vi "OCR_OCR.vi"(8 "Error":errorcluster, 11 "Image Data":T4) -> (0 "Error Out":errorcluster, 2 "Status Of Each Line Out":bool[](array[boolean]), 3 "Text Out":T6[](array[typedef]), 5 "Colors Out":T7, 7 "Icon Sizing Out":T1={"Rule"=enum."Static", "Header"=TRUE, "Rows"=5, "Width"=32, "Position"=enum."MID-CTR"} {"Rows" min=1 max=5 step=1; "Width" min=7 max=32 step=1})   [LabVIEW 2009]
doc: "Extract text data from image cluster"
uses:
  Controls/Cluster/Cluster_Icon Color Set.ctl
  Controls/Enum/ENUM_Frame Template Select.ctl
  Controls/String_Picture/STRING_Line Display.ctl
  Controls/Cluster/Cluster_Image Data.ctl
  Controls/Cluster/CLuster_Selectoin Box.ctl
  Controls/Cluster/Cluster_Sizing Data.ctl
  Controls/Enum/ENUM_Icon Sizing.ctl
  Controls/Enum/RBENUM_Icon Position.ctl
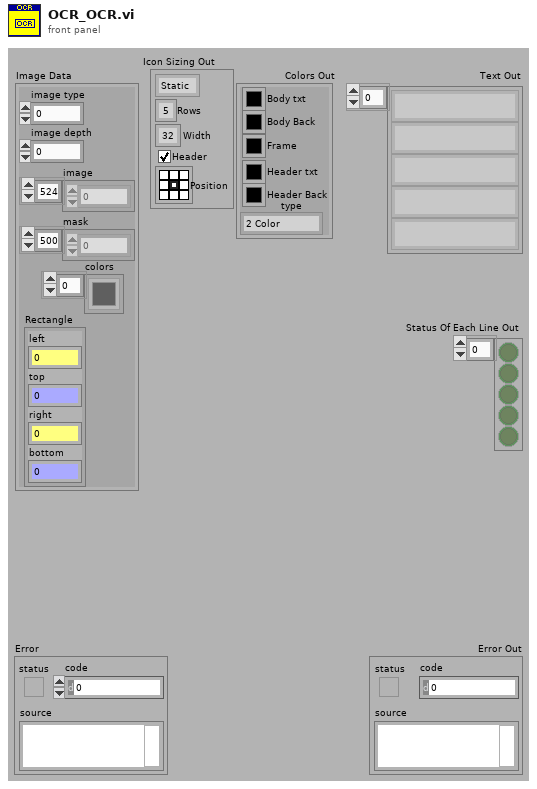
[diagram p1: front panel]
types:
  T1 = typedef "Cluster_Sizing Data.ctl" = cluster{"Rule":T2, "Header":bool, "Rows":u32, "Width":u32, "Position":T3}
  T2 = typedef "ENUM_Icon Sizing.ctl" = enum16{"Static", "Auto"}
  T3 = typedef "RBENUM_Icon Position.ctl" = enum32{"LFT-TOP", "MID-TOP", "RGT-TOP", "LFT-CTR", "MID-CTR", "RGT-CTR", "LFT-BOT", "MID-BOT", "RGT-BOT"}
  T4 = typedef "Cluster_Image Data.ctl" = cluster{"image type":i32, "image depth":i32, "image":u8[], "mask":u8[], "colors":u32[], "Rectangle":T5}
  T5 = typedef "CLuster_Selectoin Box.ctl" = cluster{"left":i16, "top":i16, "right":i16, "bottom":i16}
  T6 = typedef "STRING_Line Display.ctl" = string
  T7 = typedef "Cluster_Icon Color Set.ctl" = cluster{"Body txt":u32, "Body Back":u32, "Frame":u32, "Header txt":u32, "Header Back":u32, "type":T8}
  T8 = typedef "ENUM_Frame Template Select.ctl" = enum16{"2 Color", "5 Color"}
  T9 = typedef "imagedata.ctl" = cluster{"image type":i32, "image depth":i32, "image":u8[], "mask":u8[], "colors":u32[], "Rectangle":cluster{"left":i16, "top":i16, "right":i16, "bottom":i16}}
  T10 = typedef "Color Box Array_2D Icon Viewer.ctl" = u32[][]
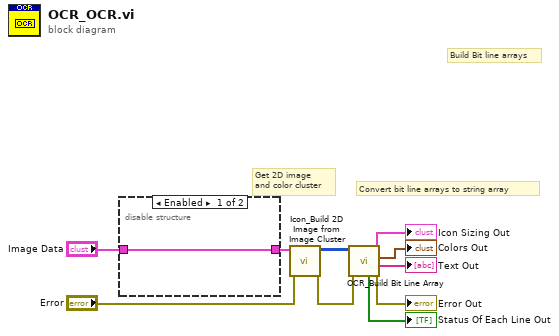
[diagram p0: block diagram]
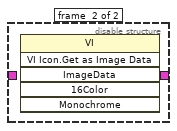
[diagram p2: hidden frame]
diagram:
  # "Convert bit line arrays to string array"
  # "Build Bit line arrays"
  # "Get 2D image\nand color cluster"
  n1 = disable-structure shown="Enabled" {
    disable-tunnel: [w11 w12] -> w9
    disable-tunnel: "Image Data" -> [w11 _]
    frame #0 {
    }
    frame #1 {
      n2 = invoke class="VI" method="VI Icon.Get as Image Data"() -> ("ImageData"=w12:T9)  [unwired: 6 in, 5 out]
    }
  }
  n3 = call "Icon_Build 2D Image from Image Cluster.vi"("Error"="Error", "Color256"=w9) -> ("Error Out"=w6:errorcluster, "2D Image Out"=w8:T10)  [unwired: 8 in]
  n4 = call "OCR_Build Bit Line Array.vi"("Error"=w6, "2D Image"=w8) -> ("Error Out"=→"Error Out":errorcluster, "Text Out"=→"Text Out":T6[], "Colors Out"=→"Colors Out":T7, "Format Out"=→"Icon Sizing Out":T1, "Status Of Each Line Out"=→"Status Of Each Line Out":bool[])  [unwired: 5 in]
